vi "_TangoReloadDeviceInterface.vi"(1 "error in":errorcluster, 2 "device name":string) -> (0 "error out":errorcluster)   [LabVIEW 2014, in "tango.lvlib"]
uses:
  tango.lvlib
  tango_binding.so
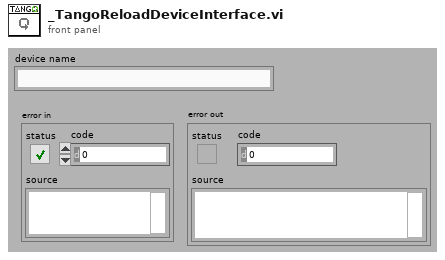
[diagram p1: front panel]
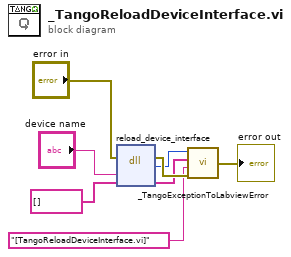
[diagram p0: block diagram]
diagram:
  n1 = dll-call lib="tango_binding.*" fn="reload_device_interface"(error in="error in", "dev_name"="device name", "error_stack"=string[] [] ("Error Stack")) -> (error out=w5:errorcluster, "return type"=w4:i32, "error_stack"=w3:string[])  [unwired: 3 in, 1 out]
  n2 = call "_TangoExceptionToLabviewError.vi"("error in"=w5, "location"="[TangoReloadDeviceInterface.vi]", "error stack"=w3, "error code"=w4) -> ("error out"=→"error out":errorcluster)
